vi "Teardown.vi"(11 "jettl in":refnum<class "jettl.lvclass">) -> (2 "Teardown?":bool, 3 "jettl out":refnum<class "jettl.lvclass">)   [LabVIEW 2021, in "jettl.lvlib" / "jettl.lvclass"]
uses:
  jettl.lvclass
  C:/git/jettl/src/jettl/Actor/Actor.lvclass
  jettl.lvclass/jettl.ctl
  State/State/State.lvclass
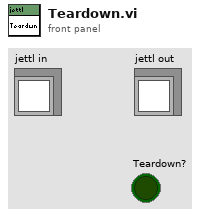
[diagram p1: front panel]
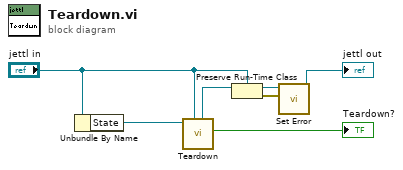
[diagram p0: block diagram]
diagram:
  n1 = Unbundle By Name("jettl in") -> ("State"=w7:refnum<class "State.lvclass">)
  n2 = call-dynamic "Teardown.vi"("Actor in"="jettl in", "State in"=w7) -> ("Teardown?"=→"Teardown?":bool, "Actor out"=w4:refnum<class "Actor.lvclass">)  [unwired: 8 in]
  n3 = Preserve Run-Time Class(object in=w4, 2:"jettl in") -> (object out=w3:refnum<class "jettl.lvclass">, error out=w1:errorcluster)  [unwired: 1 in]
  n4 = call-dynamic "Set Error.vi"("Error"=w1, "jettl in"=w3) -> ("jettl out"=→"jettl out":refnum<class "jettl.lvclass">)  [unwired: 9 in]
